vi "DeviceOff.vi"(8 "error in (no error)":errorcluster, 11 "NhRegenGridSim in":refnum<class "NHRGridSim.lvclass">) -> (0 "error out":errorcluster, 3 "NhRegenGridSim out":refnum<class "NHRGridSim.lvclass">)   [LabVIEW 2018, in "AcPwrPlugins.lvlib" / "NHRGridSim.lvclass"]
doc: "This VI (if the unit is not already off) turns off the unit. Off is defined as the output relay being open."
uses:
  NHRGridSim.lvclass
  <instrlib>/NH Research 9400 Series/NH Research 9400 Series.lvlib
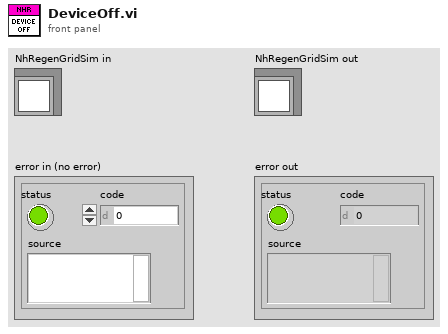
[diagram p1: front panel]
types:
  T1 = typedef "AcPwrPlugins.lvlib/NHRGridSim.lvclass/Modules.ctl" = cluster{"Measurement":cluster{"ApertureLength (s)":dbl, "NumberOfSamples":u32}, "Ranges":cluster{"Irange (A)":dbl, "Vrange (V)":dbl}, "Mode":u8, "Handle":string, "FreqOut (Hz)":dbl, "Connected":bool, "btnIdQuery":bool, "btnReset":bool, "Initialize Timeout ( ms)":u32, "Phase (0: All)":i32, "WatchDog":cluster{"Enable WatchDog":bool, "Robust WatchDog":bool, "Watchdog Interval (s)":dbl}, "Safety Limits":cluster{"Min Voltage (V)":dbl, "Min Voltage Time (s)":dbl, "Max Voltage (V)":dbl, "MaxVoltage Time (s)":dbl, "Max Source Amps (A)":dbl, "Max Source Amps Time (s)":dbl, "Max Sink Amps (A)":dbl, "Max Sink Amps Time (s)":dbl, "Max Source Power (W)":dbl, "Max Source Power Time (s)":dbl, "Max Sink Power (W)":dbl, "Max Sink Power Time (s)":dbl, "Peak Voltage (V)":dbl, "Peak Voltage Enable":bool, "Peak Amps (A)":dbl, "Peak Amps Enable":bool}, "Phases":cluster{"Pout (W)":dbl, "Iout (A)":dbl, "PhaseAngle":dbl, "Vout (V)":dbl, "Phase Name":string}[], "Regulation Gain":dbl, "ChangeOntheFly":bool, "Synchronize Output \nto Phase":bool, "Slew Rate":cluster{"Voltage Slew (Volts/s)":dbl, "Phase Angle (Degrees/s)":dbl}}[]
  T2 = cluster{"Pout (W)":dbl, "Iout (A)":dbl, "PhaseAngle":dbl, "Vout (V)":dbl, "Phase Name":string}[]
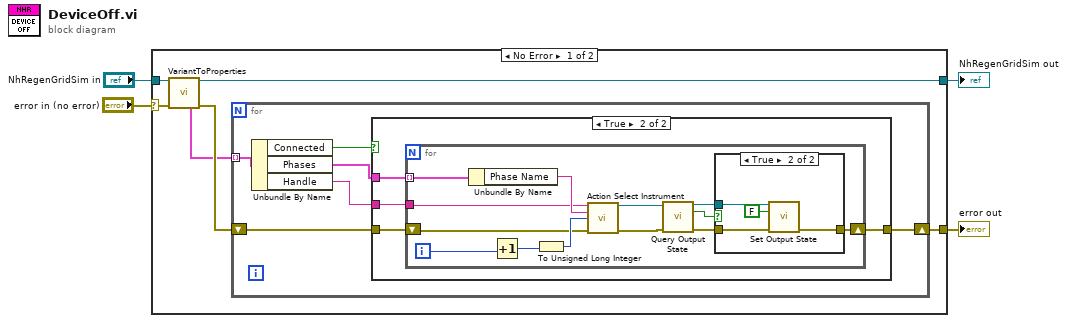
[diagram p0: block diagram]
diagram:
  n1 = case shown="No Error" "error in (no error)" {
    selector: "error in (no error)" -> [w8 w40]
    tunnel: [w10 w40] -> w4
    tunnel: [w7 w39] -> w3
    tunnel: "NhRegenGridSim in" -> [w9 w39]
    frame No Error {
      n2 = call "VariantToProperties.vi"("NHRGridSim in"=w9, "error in (no error)"=w8) -> ("NHRGridSim out"=w7:refnum<class "NHRGridSim.lvclass">, "Modules"=w5:T1, "error out"=w6:errorcluster)  [unwired: 7 in, 4 out]
      n3 = for {
        tunnel: w5 -> [w16] mode=indexing
        shift-right: [w14] -> w10
        shift-left: w6 -> [w15]
        n4 = Unbundle By Name(w16) -> ("Connected"=w13:bool, "Phases"=w11:T2, "Handle"=w12:string)
        n5 = case shown="True" w13 {
          tunnel: w15 -> [w17 w21]
          tunnel: [w17 w20] -> w14
          tunnel: w12 -> [_ w19]
          tunnel: w11 -> [_ w18]
          frame False {
          }
          frame True {
            n6 = for {
              tunnel: w19 -> [w26]
              shift-right: [w31] -> w20
              shift-left: w21 -> [w25]
              tunnel: w18 -> [w23] mode=indexing
              i -> [w24]
              n7 = Unbundle By Name(w23) -> ("Phase Name"=w27:string)
              n8 = Increment(x=w24) -> (x+1=w28:i32)
              n9 = To Unsigned Long Integer(number=w28) -> (unsigned 32bit integer=w29:u32)
              n10 = call <instrlib>:"Action Select Instrument.vi"("VISA resource name"=w26, "Logical Instrument Name"=w27, "Logical Instrument Number"=w29, "error in (no error)"=w25) -> ("VISA resource name out"=w22:refnum<visa-resource-name>)  [unwired: 10 in, 1 out]
              n11 = call <instrlib>:"Query Output State.vi"("VISA resource name"=w22, "error in (no error)"=w25) -> ("VISA resource name out"=w30:refnum<visa-resource-name>, "Output Enabled"=w33:bool, "error out"=w32:errorcluster)  [unwired: 11 in]
              n12 = case shown="True" w33 {
                tunnel: w32 -> [w34 w38]
                tunnel: [w34 w37] -> w31
                tunnel: w30 -> [_ w36]
                frame False {
                }
                frame True {
                  n13 = call <instrlib>:"Set Output State.vi"("VISA resource name"=w36, "Output State (F: Disable)"=FALSE, "error in (no error)"=w38) -> ("error out"=w37:errorcluster)  [unwired: 11 in, 1 out]
                }
              }
            }
          }
        }
      }
    }
    frame Error {
    }
  }
  "error out" <- w4
  "NhRegenGridSim out" <- w3
